vi "SVT Crosstalk.vi"   [LabVIEW 2017, in "SoundVib_SingleTone.lvlib"]
doc: "Computes the crosstalk between <B>stimulus signal X</B> and <B>idle-channel response signal Y</B> to a response signal at the fundamental frequency. This VI returns the detected tone stimulus, detected tone idle-channel response, and crosstalk. This VI does not maintain state internally; you can use this VI in a loop to process multiple blocks. Wire data to the <B> stimulus signal X</B> and <B>idle-channel response signal Y</B> inputs to determine the polymorphic instance to use or manually select the instance."
uses:
  <vilib>/addons/Sound and Vibration/svt_Single Tone Measurements/SoundVib_SingleTone.lvlib
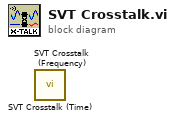
[diagram p0: block diagram]
diagram:
  n1 = call <vilib>:"SVT Crosstalk (Time).vi"() -> ()  [unwired: 12 in, 8 out]
  n2 = call <vilib>:"SVT Crosstalk (Frequency).vi"() -> ()  [unwired: 12 in, 8 out]
